vi "SubVI Terminals Info.vi"(8 "error in":errorcluster, 11 "SubVI ref":refnum<vi>) -> (0 "error out":errorcluster, 3 "output cluster":T1)   [LabVIEW 2014]
doc: "Convert string ClassName into specific reference ie. Terminal owner which will be SubVI converts this VI to ref.to SubVI so we caqn easily create property and ivnoke methods."
uses:
  <vilib>/regexp/Match Regular Expression.xnode
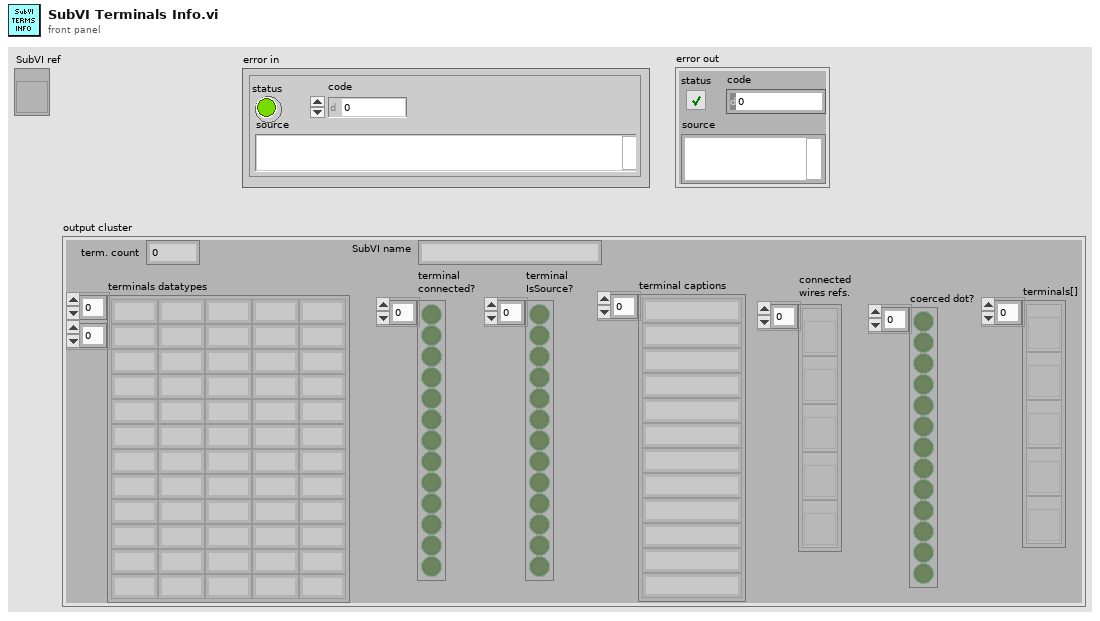
[diagram p1: front panel]
types:
  T1 = cluster{"terminals datatypes":string[][], "terminal\nconnected?":bool[], "terminal captions":string[], "term. count":i32, "terminal\nIsSource?":bool[], "SubVI name":string, "connected\nwires refs.":refnum<vi>[], "coerced dot?":bool[], "terminals[]":refnum<vi>[]}
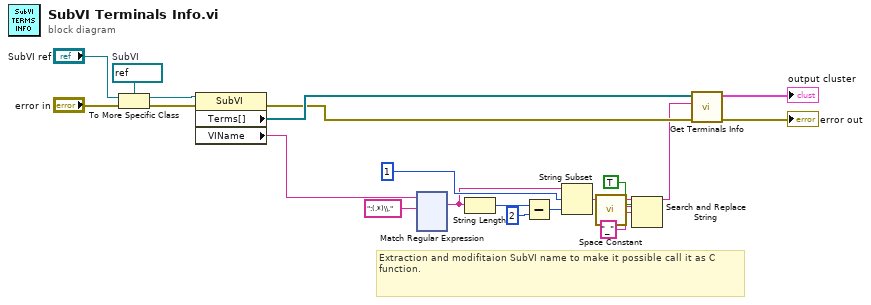
[diagram p0: block diagram]
diagram:
  w21 = refnum<vi> refnum  # SubVI
  # "Extraction and modifitaion SubVI name to make it possible call it as C function."
  n1 = To More Specific Class(target class=w21, reference="SubVI ref", error in="error in") -> (specific class reference=w18:refnum<vi>, error out=w17:errorcluster)
  n2 = property class="SubVI"(reference=w18, error in=w17) -> (error out=w4:errorcluster, "Terms[]"=w5:refnum<vi>[], "VIName"=w6:string)  [unwired: 1 out]
  n3 = xnode "Match Regular Expression"("input string"=w6, "regular expression"=":(.*)\\.") -> ("whole match"=w12:string)  [unwired: 4 in, 4 out]
  n4 = String Length(string=w12) -> (length=w14:i32)
  n5 = Subtract(x=w14, y=2 ("offset (0)")) -> (x-y=w11:i32)
  n6 = String Subset(string=w12, offset (0)=1, length (rest)=w11) -> (substring=w10:string)
  n7 = call <vilib>:"Space Constant.vi"() -> ("String"=w9:string)
  n8 = Search and Replace String(replace all?=TRUE ("replace all? (F)"), input string=w10, search string=w9, replace string="_" ("replace string (\"\")")) -> (result string=w3:string)  [unwired: 4 in, 3 out]
  n9 = call "Get Terminals Info.vi"("error in (no error)"=w4, "structure name"=w3, "Terms[]"=w5) -> ("error out"=→"error out":errorcluster, "output cluster"=→"output cluster":T1)  [unwired: 7 in]
